vi "Initialize.vi"(8 "error in":errorcluster, 10 "parameters":variant, 11 "node in":refnum<class "NISE_CEF_Node.lvclass">) -> (0 "error out":errorcluster, 2 "summary":T2[](array[typedef]), 3 "data value reference":T1)   [LabVIEW 2014, in "NISE_CEF_Node.lvclass"]
doc: "Initializes the data of a node to its default state.\nThe object is not created inside of this VI, because it is created from a File depending on user selection."
uses:
  NISE_CEF_Node.lvclass
  Summary.ctl
  NodeRef.ctl
  NISE_CEF_TreeControl.lvlib
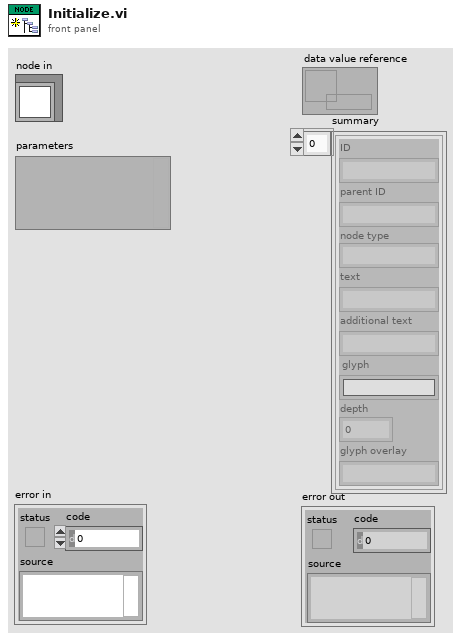
[diagram p1: front panel]
types:
  T1 = typedef "NISE_CEF_Node.lvclass/NodeRef.ctl" = refnum<data-value>
  T2 = typedef "NISE_CEF_Node.lvclass/Summary.ctl" = cluster{"ID":string, "parent ID":string, "node type":string, "text":string, "additional text":string, "glyph":string, "depth":i32, "glyph overlay":string}
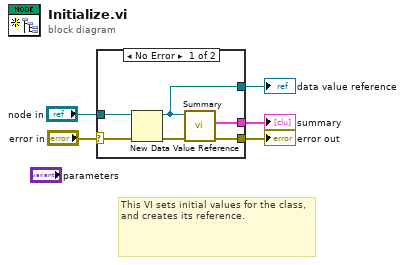
[diagram p0: block diagram]
diagram:
  # "This VI sets initial values for the class, and creates its reference."
  n1 = case shown="No Error" "error in" {
    selector: "error in" -> [w6 w12]
    tunnel: [w11 w12] -> w4
    tunnel: [w8 _] -> w1
    tunnel: "node in" -> [w7 _]
    tunnel: [w10 _] -> w2
    frame No Error {
      n2 = New Data Value Reference(data value=w7, error in=w6) -> (data value reference=w8:refnum<data-value>, error out=w9:errorcluster)
      n3 = call "Summary.vi"("error in"=w9, "node self ref"=w8) -> ("error out"=w11:errorcluster, "summary"=w10:T2[])  [unwired: 8 in]
    }
    frame Error {
    }
  }
  "error out" <- w4
  "summary" <- w2
  "data value reference" <- w1
